vi "Save DAC Configuration.vi"(8 "error in":errorcluster, 10 "Config File refnum in":T1, 11 "DAC LN2 Temp in":refnum<class "DAC LN2 Temp.lvclass">) -> (0 "error out":errorcluster, 2 "Config File refnum out":T1, 3 "DAC LN2 Temp out":refnum<class "DAC LN2 Temp.lvclass">)   [LabVIEW 2019, in "DAC.lvlib" / "DAC LN2 Temp.lvclass"]
uses:
  DAC LN2 Temp.lvclass
  C:/Users/krio/Documents/LV_Projects/test-stand/App/DAC/DAC.lvclass
  <vilib>/Utility/config.llb/Config Data RefNum.ctl
  DAC.lvclass/DAC.ctl
  DAC LN2 Temp.lvclass/DAC LN2 Temp.ctl
  <vilib>/Utility/config.llb/Write Key (String).vi
  <vilib>/Utility/config.llb/Write Key (Double).vi
  DAC.lvclass
  <vilib>/Utility/config.llb/NI_LVConfig.lvlib
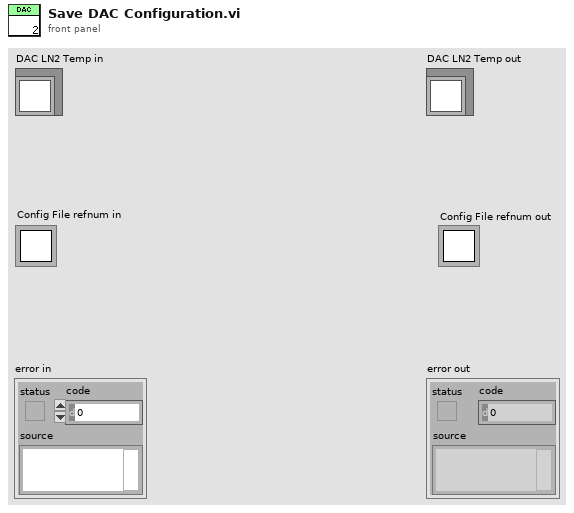
[diagram p1: front panel]
types:
  T1 = typedef "NI_LVConfig.lvlib/Config Data RefNum.ctl" = refnum<k1>
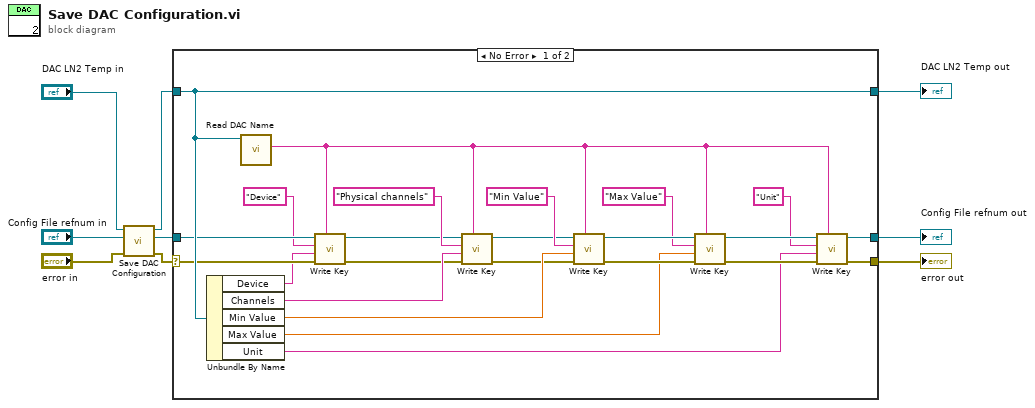
[diagram p0: block diagram]
diagram:
  n1 = call-parent "Save DAC Configuration.vi"("error in"="error in", "Config File refnum in"="Config File refnum in", "DAC in"="DAC LN2 Temp in") -> ("error out"=w4:errorcluster, "Config File refnum out"=w5:T1, "DAC out"=w6:refnum<class "DAC LN2 Temp.lvclass">)  [unwired: 6 in]
  n2 = case shown="No Error" w4 {
    selector: w4 -> [w15 w36]
    tunnel: [w26 w36] -> w1
    tunnel: [w21 w35] -> w3
    tunnel: w6 -> [w21 w35]
    tunnel: w5 -> [w16 w34]
    tunnel: [w25 w34] -> w2
    frame No Error {
      n3 = Unbundle By Name(w21) -> ("Device"=w11:string, "Channels"=w17:string, "Min Value"=w24:dbl, "Max Value"=w23:dbl, "Unit"=w22:string)
      n4 = call "Read DAC Name.vi"("DAC in"=w21) -> ("DAC Name"=w10:string)  [unwired: 8 in, 2 out]
      n5 = call-poly <vilib>:"Write Key.vi"("section"=w10, "error in (no error)"=w15, "value"=w11, "key"="Device", "refnum"=w16) -> ("error out"=w13:errorcluster, "refnum out"=w14:T1)  [unwired: 4 in, 1 out]
      n6 = call-poly <vilib>:"Write Key.vi"("section"=w10, "error in (no error)"=w13, "value"=w17, "key"="Physical channels", "refnum"=w14) -> ("error out"=w19:errorcluster, "refnum out"=w20:T1)  [unwired: 4 in, 1 out]
      n7 = call-poly <vilib>:"Write Key.vi"("section"=w10, "error in (no error)"=w19, "value"=w24, "key"="Min Value", "refnum"=w20) -> ("error out"=w31:errorcluster, "refnum out"=w33:T1)  [unwired: 4 in, 1 out]
      n8 = call-poly <vilib>:"Write Key.vi"("section"=w10, "error in (no error)"=w31, "value"=w23, "key"="Max Value", "refnum"=w33) -> ("error out"=w30:errorcluster, "refnum out"=w32:T1)  [unwired: 4 in, 1 out]
      n9 = call-poly <vilib>:"Write Key.vi"("section"=w10, "error in (no error)"=w30, "value"=w22, "key"="Unit", "refnum"=w32) -> ("error out"=w26:errorcluster, "refnum out"=w25:T1)  [unwired: 4 in, 1 out]
    }
    frame Error {
    }
  }
  "error out" <- w1
  "DAC LN2 Temp out" <- w3
  "Config File refnum out" <- w2
